vi "InspectTell.vi"(7 "ConcreteActor":refnum<class "ConcreteActor.lvclass">, 10 "ActorAlias":string, 11 "Message":refnum<class "Message.lvclass">) -> (3 "Message":refnum<class "Message.lvclass">, 5 "ConcreteActor":refnum<class "ConcreteActor.lvclass">)   [LabVIEW 2020, in "_Template.lvlib" / "ActorTemplate.lvlib" / "{{Name}}.lvlib" / "ConcreteActor.lvclass"]
uses:
  ConcreteActor.lvclass
  jettl/jettl/Message/Message.lvclass
  ConcreteActor.lvclass/ConcreteActor.ctl
  jettl/jettl/Actor/Actor.lvclass
panel:
  # "This front panel should not be manipulated."
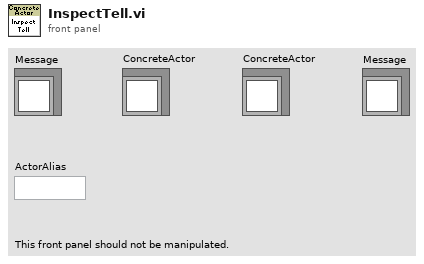
[diagram p1: front panel]
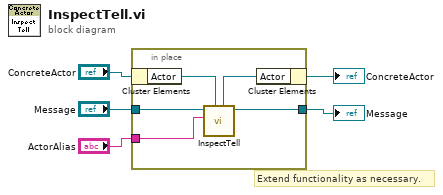
[diagram p0: block diagram]
diagram:
  # "Extend functionality as necessary."
  n1 = in-place {
    in-place-border: "ActorAlias" -> [w6]
    in-place-border: [w8] -> w2
    in-place-border: "Message" -> [w7]
    n2 = in-place-cluster #1("ConcreteActor") -> ("Actor"=w10:refnum<class "Actor.lvclass">)
    n3 = call-dynamic "InspectTell.vi"("Actor"=w10, "ActorAlias"=w6, "Message"=w7) -> ("Message"=w8:refnum<class "Message.lvclass">, "Actor"=w9:refnum<class "Actor.lvclass">)  [unwired: 7 in]
    n4 = in-place-cluster #1("Actor"=w9) -> (→"ConcreteActor":refnum<class "ConcreteActor.lvclass">)
  }
  "Message" <- w2
